vi "Restore Data Store Paths.vi"(8 "error in":errorcluster, 11 "original values":T1) -> (0 "error out":errorcluster)   [LabVIEW 2024]
uses:
  Environment Values.ctl
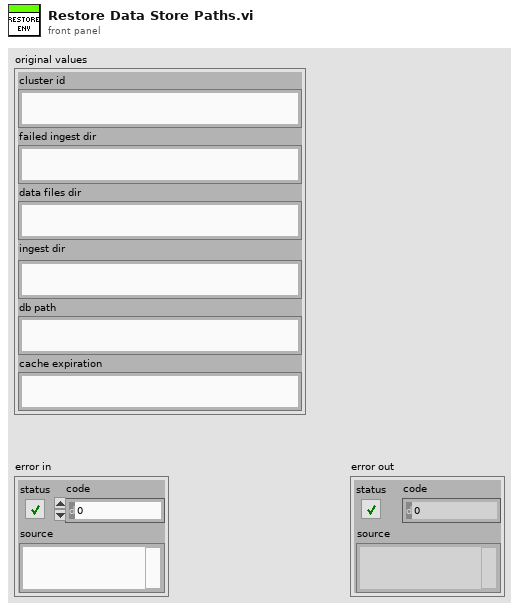
[diagram p1: front panel]
types:
  T1 = typedef "Environment Values.ctl" = cluster{"cluster id":string, "failed ingest dir":string, "data files dir":string, "ingest dir":string, "db path":string, "cache expiration":string}
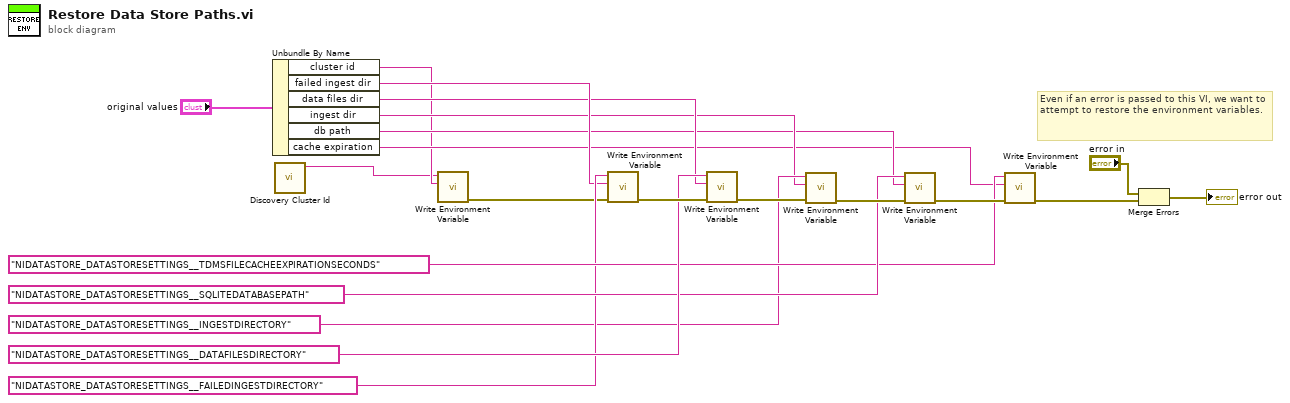
[diagram p0: block diagram]
diagram:
  # "Even if an error is passed to this VI, we want to attempt to restore the environment variables."
  n1 = Unbundle By Name("original values") -> ("cluster id"=w5:string, "failed ingest dir"=w11:string, "data files dir"=w10:string, "ingest dir"=w9:string, "db path"=w8:string, "cache expiration"=w7:string)
  n2 = call "Discovery Cluster Id.vi"() -> ("nidiscovery_clusterid"=w4:string)  [unwired: 11 in]
  n3 = call "Write Environment Variable.vi"("value"=w5, "name"=w4) -> ("error out"=w6:errorcluster)  [unwired: 9 in]
  n4 = call "Write Environment Variable.vi"("error in"=w6, "value"=w11, "name"="NIDATASTORE_DATASTORESETTINGS__FAILEDINGESTDIRECTORY") -> ("error out"=w21:errorcluster)  [unwired: 8 in]
  n5 = call "Write Environment Variable.vi"("error in"=w21, "value"=w10, "name"="NIDATASTORE_DATASTORESETTINGS__DATAFILESDIRECTORY") -> ("error out"=w20:errorcluster)  [unwired: 8 in]
  n6 = call "Write Environment Variable.vi"("error in"=w20, "value"=w9, "name"="NIDATASTORE_DATASTORESETTINGS__INGESTDIRECTORY") -> ("error out"=w19:errorcluster)  [unwired: 8 in]
  n7 = call "Write Environment Variable.vi"("error in"=w19, "value"=w8, "name"="NIDATASTORE_DATASTORESETTINGS__SQLITEDATABASEPATH") -> ("error out"=w18:errorcluster)  [unwired: 8 in]
  n8 = call "Write Environment Variable.vi"("error in"=w18, "value"=w7, "name"="NIDATASTORE_DATASTORESETTINGS__TDMSFILECACHEEXPIRATIONSECONDS") -> ("error out"=w2:errorcluster)  [unwired: 8 in]
  n9 = Merge Errors("error in", w2) -> (→"error out":errorcluster)
